vi "JG_guanli.vi"(3 "key":string, 6 "caozuo":string, 7 "LabVIEW Web Service Request":refnum<class "Web Request.lvclass"> caption="LabVIEW Web服务请求", 8 "name":string, 9 "number":string, 10 "id":string, 11 "action":string) -> (0 "error":errorcluster)   [LabVIEW 2017]
uses:
  <vilib>/wsapi/Web Request.lvclass
panel:
  out "postdata":string caption="post数据"
  out "error out":errorcluster caption="错误输出"
  # "Web服务请求输入接线端用于调用“Web服务”选板的VI。除非不需要访问该选板，否则不要在连线板上删除这个输入接线端。"
  # "添加至连线板的每一个其他输入控件，在URL中对应于一个输入。如需在接线端模式输出（默认设置）下包含显示控件，则该显示控件必须与连线板相连。"
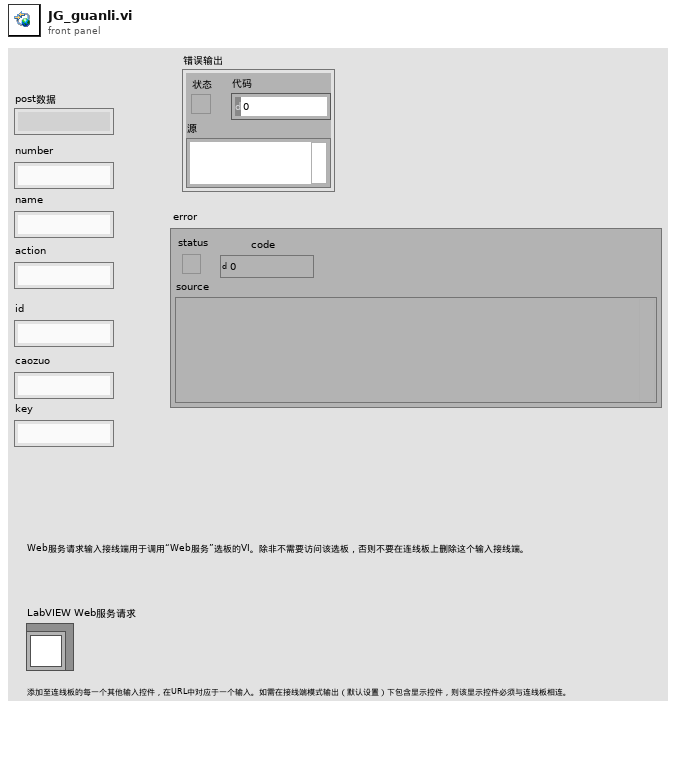
[diagram p1: front panel]
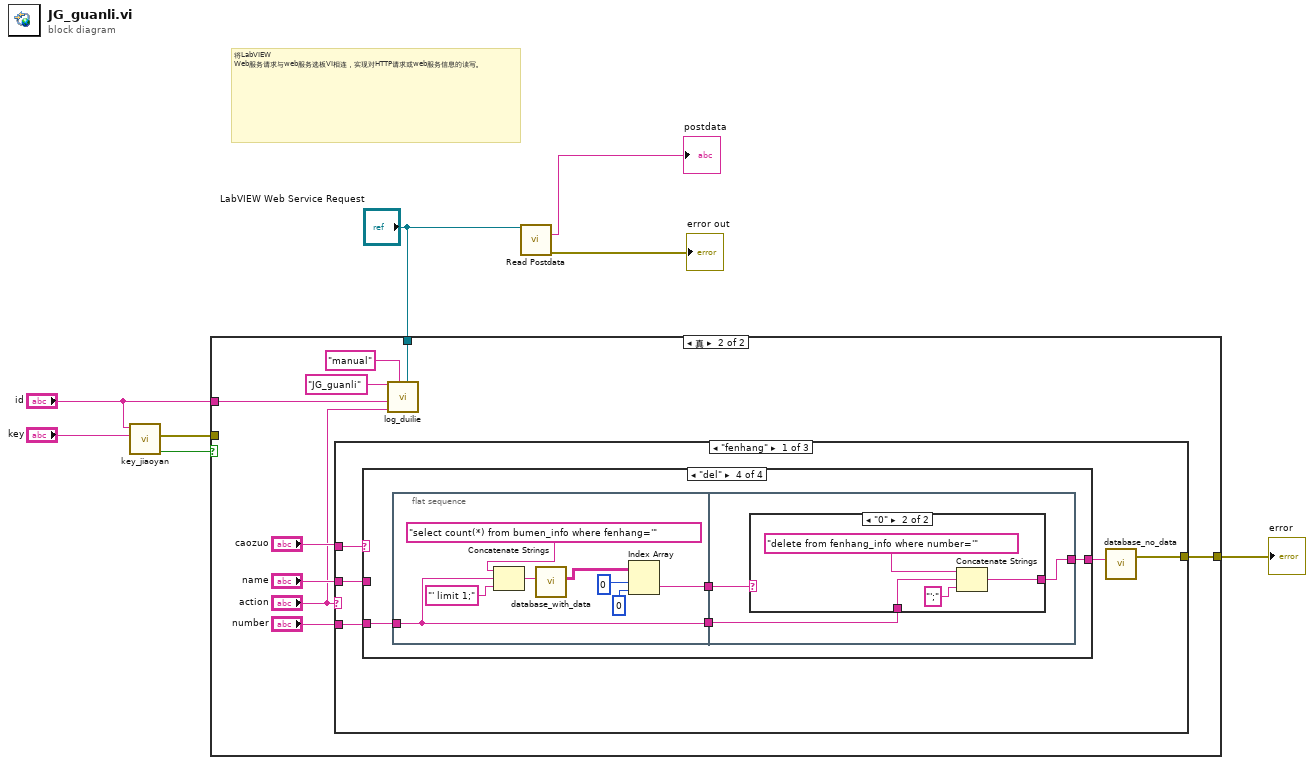
[diagram p0: block diagram]
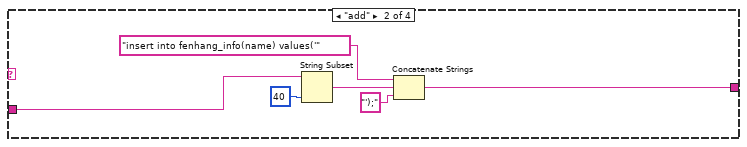
[diagram p4: hidden frame]
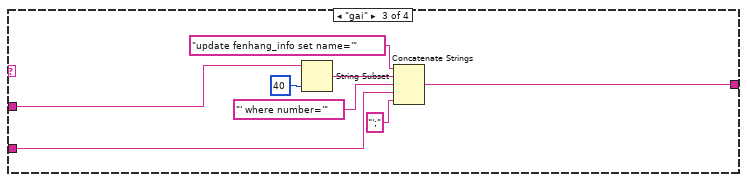
[diagram p5: hidden frame]
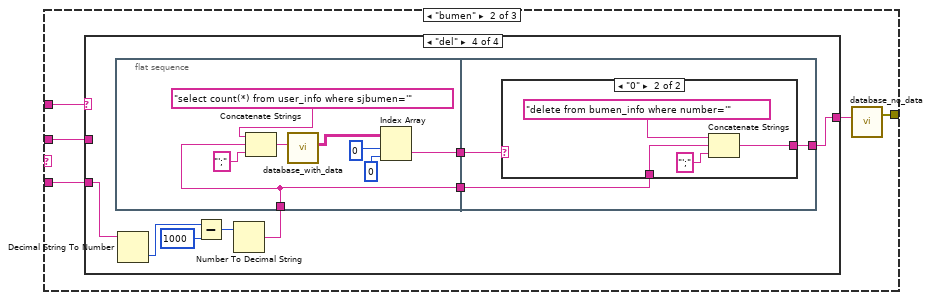
[diagram p7: hidden frame]
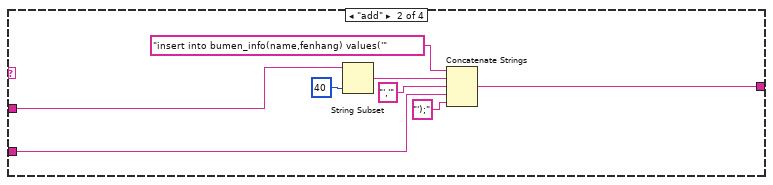
[diagram p9: hidden frame]
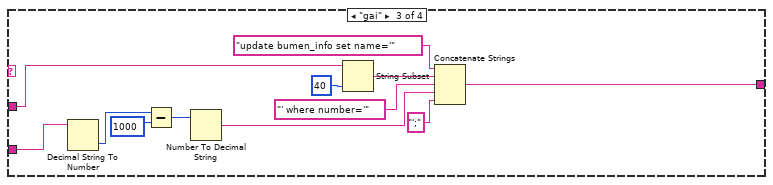
[diagram p10: hidden frame]
diagram:
  # "将LabVIEW Web服务请求与web服务选板VI相连，实现对HTTP请求或web服务信息的读写。"
  n1 = call "key_jiaoyan.vi"("key_client"="key", "gonghao"="id") -> ("jy"=w2:bool, "error"=w1:errorcluster)  [unwired: 8 in]
  n2 = case shown="真" w2 {
    tunnel: [w9 w18] -> w7
    tunnel: "LabVIEW Web Service Request" -> [_ w14]
    tunnel: "id" -> [_ w10]
    tunnel: w1 -> [w9 _]
    frame False {
    }
    frame True {
      n3 = case shown="\"fenhang\"" "action" {
        tunnel: [w22 w60 _] -> w18
        tunnel: "caozuo" -> [w21 w59 _]
        tunnel: "name" -> [w20 w58 _]
        tunnel: "number" -> [w19 w57 _]
        frame "fenhang" {
          n4 = case shown="\"del\"" w21 {
            tunnel: [_ w25 w33 w41] -> w23
            tunnel: w20 -> [_ w24 w32 _]
            tunnel: w19 -> [_ _ w30 w40]
            frame "假", Default {
            }
            frame "add" {
              n5 = String Subset(string=w24, length (rest)=40 ("长度（剩余）")) -> (substring=w28:string)  [unwired: 1 in]
              n6 = Concatenate Strings("insert into fenhang_info(name) values('" ("格式字符串"), w28, "');" ("字符串")) -> (w25:string)
            }
            frame "gai" {
              n7 = String Subset(string=w32, length (rest)=40 ("长度（剩余）")) -> (substring=w36:string)  [unwired: 1 in]
              n8 = Concatenate Strings("update fenhang_info set name='" ("格式字符串"), w36, "' where number='" ("字符串"), w30, "';" ("字符串")) -> (w33:string)
            }
            frame "del" {
              n9 = flat-sequence {
                tunnel: w40 -> [w47]
                tunnel: [w47] -> w39
                tunnel: [w42] -> w38
                tunnel: [w52] -> w41
                tunnel: w39 -> [w51]
                tunnel: w38 -> [w50]
                frame #0 {
                  n10 = Concatenate Strings("select count(*) from bumen_info where fenhang='" ("格式字符串"), w47, "' limit 1;" ("字符串")) -> (w46:string)
                  n11 = call "database_with_data.vi"("input"=w46) -> ("Data"=w43:string[][])  [unwired: 9 in, 1 out]
                  n12 = Index Array(array=w43, index (row)=0 ("索引 (行)"), index (col)=0 ("禁用的索引 (列)")) -> (element=w42:string)
                }
                frame #1 {
                  n13 = case shown="\"0\"" w50 {
                    tunnel: [_ w54] -> w52
                    tunnel: w51 -> [_ w53]
                    frame "假", Default {
                    }
                    frame "0" {
                      n14 = Concatenate Strings("delete from fenhang_info where number='" ("格式字符串"), w53, "';" ("字符串")) -> (w54:string)
                    }
                  }
                }
              }
            }
          }
          n15 = call "database_no_data.vi"("input"=w23) -> ("error"=w22:errorcluster)  [unwired: 2 in]
        }
        frame "bumen" {
          n16 = case shown="\"del\"" w59 {
            tunnel: [_ w66 w77 w83] -> w61
            tunnel: w58 -> [_ w65 w76 _]
            tunnel: w57 -> [_ w63 w74 w82]
            frame "假", Default {
            }
            frame "add" {
              n17 = String Subset(string=w65, length (rest)=40 ("长度（剩余）")) -> (substring=w68:string)  [unwired: 1 in]
              n18 = Concatenate Strings("insert into bumen_info(name,fenhang) values('" ("格式字符串"), w68, "','" ("字符串"), w63, "');" ("字符串")) -> (w66:string)
            }
            frame "gai" {
              n19 = Decimal String To Number(string=w74) -> (number=w73:i32)  [unwired: 2 in, 1 out]
              n20 = Subtract(x=w73, y=1000) -> (x-y=w71:i32)
              n21 = Number To Decimal String(number=w71) -> (decimal integer string=w70:string)  [unwired: 1 in]
              n22 = String Subset(string=w76, length (rest)=40 ("长度（剩余）")) -> (substring=w80:string)  [unwired: 1 in]
              n23 = Concatenate Strings("update bumen_info set name='" ("格式字符串"), w80, "' where number='" ("字符串"), w70, "';" ("字符串")) -> (w77:string)
            }
            frame "del" {
              n24 = flat-sequence {
                tunnel: w87 -> [w95]
                tunnel: [w95] -> w89
                tunnel: [w90] -> w88
                tunnel: [w100] -> w83
                tunnel: w89 -> [w99]
                tunnel: w88 -> [w98]
                frame #0 {
                  n25 = Concatenate Strings("select count(*) from user_info where sjbumen='" ("格式字符串"), w95, "';" ("字符串")) -> (w94:string)
                  n26 = call "database_with_data.vi"("input"=w94) -> ("Data"=w91:string[][])  [unwired: 9 in, 1 out]
                  n27 = Index Array(array=w91, index (row)=0 ("索引 (行)"), index (col)=0 ("禁用的索引 (列)")) -> (element=w90:string)
                }
                frame #1 {
                  n28 = case shown="\"0\"" w98 {
                    tunnel: [_ w102] -> w100
                    tunnel: w99 -> [_ w101]
                    frame "假", Default {
                    }
                    frame "0" {
                      n29 = Concatenate Strings("delete from bumen_info where number='" ("格式字符串"), w101, "';" ("字符串")) -> (w102:string)
                    }
                  }
                }
              }
              n30 = Decimal String To Number(string=w82) -> (number=w85:i32)  [unwired: 2 in, 1 out]
              n31 = Subtract(x=w85, y=1000) -> (x-y=w86:i32)
              n32 = Number To Decimal String(number=w86) -> (decimal integer string=w87:string)  [unwired: 1 in]
            }
          }
          n33 = call "database_no_data.vi"("input"=w61) -> ("error"=w60:errorcluster)  [unwired: 2 in]
        }
        frame Default {
        }
      }
      n34 = call "log_duilie.vi"("LabVIEW Web Service Request"=w14, "type"="manual", "action"="action", "user"=w10, "yw"="JG_guanli") -> ()  [unwired: 7 in]
    }
  }
  "error" <- w7
  n35 = call <vilib>:"Read Postdata.vi"("LabVIEW Web Service Request"="LabVIEW Web Service Request") -> ("postdata"=→"postdata":string, "error out"=→"error out":errorcluster)  [unwired: 12 in, 1 out]
